vi "Status Message.vi"(8 "Error In":errorcluster) -> (0 "Error Out":errorcluster)   [LabVIEW 2017, in "Tests.lvlib" / "Writer.lvlib"]
uses:
  Writer.lvlib
  src/LabPack/Public/Writer/Writer.lvclass/Writer.ctl
  src/LabPack/Public/Writer/Writer.lvclass
  <vilib>/addons/_JKI Toolkits/Caraya/classes/Test/Test.lvclass
  <vilib>/addons/_JKI Toolkits/Caraya/classes/Assert/Assert.lvclass
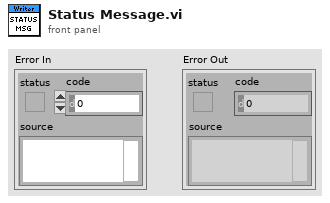
[diagram p1: front panel]
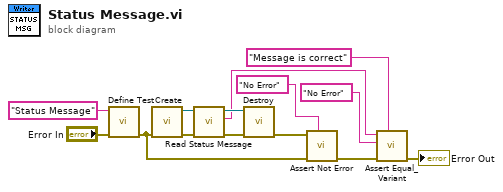
[diagram p0: block diagram]
diagram:
  n1 = call <vilib>:"Define Test.vi"("error in (no error)"="Error In", "Label (VI Title)"="Status Message") -> ("error out"=w10:errorcluster)  [unwired: 9 in]
  n2 = call "Create.vi"("Error In"=w10) -> ("Error Out"=w5:errorcluster, "Writer"=w8:refnum<class "Writer.lvclass">)  [unwired: 9 in]
  n3 = call "Read Status Message.vi"("Error In"=w5, "Writer In"=w8) -> ("Error Out"=w6:errorcluster, "Message"=w3:string, "Writer Out"=w7:refnum<class "Writer.lvclass">)  [unwired: 7 in]
  n4 = call "Destroy.vi"("Error In"=w6, "Writer"=w7) -> ("Error Out"=w9:errorcluster)  [unwired: 9 in]
  n5 = call <vilib>:"Assert Not Error.vi"("Label"="No Error", "error in (no error)"=w10, "Not Error?"=w9) -> ("error out"=w12:errorcluster)  [unwired: 8 in]
  n6 = call <vilib>:"Assert Equal_Variant.vi"("Label"="Message is correct", "error in (no error)"=w12, "Y"="No Error" ("Message"), "X"=w3) -> ("error out"=→"Error Out":errorcluster)  [unwired: 7 in]
